vi "Write Operation Complete Msg.vi"(10 "Operation Complete Msg":refnum<class "Operation Complete Msg.lvclass">, 11 "Generic Optimization in":refnum<class "Generic Optimization.lvclass">) -> (3 "Generic Optimization out":refnum<class "Generic Optimization.lvclass">)   [LabVIEW 2018, in "Generic Optimization Actor.lvlib" / "Generic Optimization.lvclass"]
uses:
  Generic Optimization.lvclass
  Generic Optimization Messages/Operation Complete Msg/Operation Complete Msg.lvclass
  Generic Optimization.lvclass/Generic Optimization.ctl
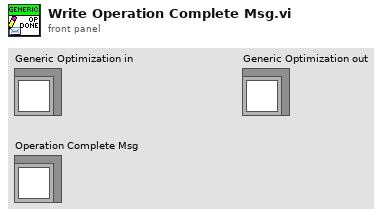
[diagram p1: front panel]
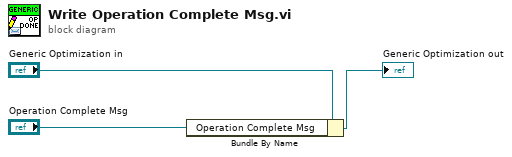
[diagram p0: block diagram]
diagram:
  n1 = Bundle By Name(cluster="Generic Optimization in", "Operation Complete Msg"="Operation Complete Msg") -> (→"Generic Optimization out":refnum<class "Generic Optimization.lvclass">)
